vi "Set Channel PWM.vi"(8 "error in (no error)":errorcluster, 9 "PWM (0-255)":u8, 10 "LED Channel (0-18, 0=all)":u8=255, 11 "LINX-SN3218 in":refnum<class "LINX-SN3218.lvclass">) -> (0 "error out":errorcluster, 3 "LINX-SN3218 out":refnum<class "LINX-SN3218.lvclass">)   [LabVIEW 2020, in "LINX-SN3218.lvclass"]
doc: "Sets the individual PWM value (0-255 = 0-100% duty cycle) for the specified channel (0-18)."
uses:
  LINX-SN3218.lvclass
  LINX I2C/LINX I2C.lvclass
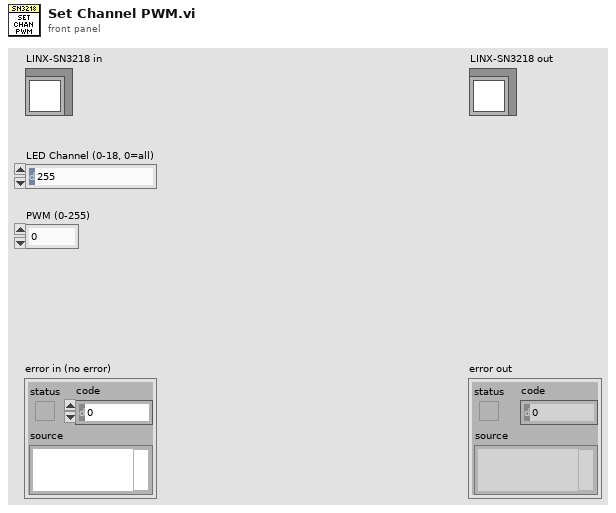
[diagram p1: front panel]
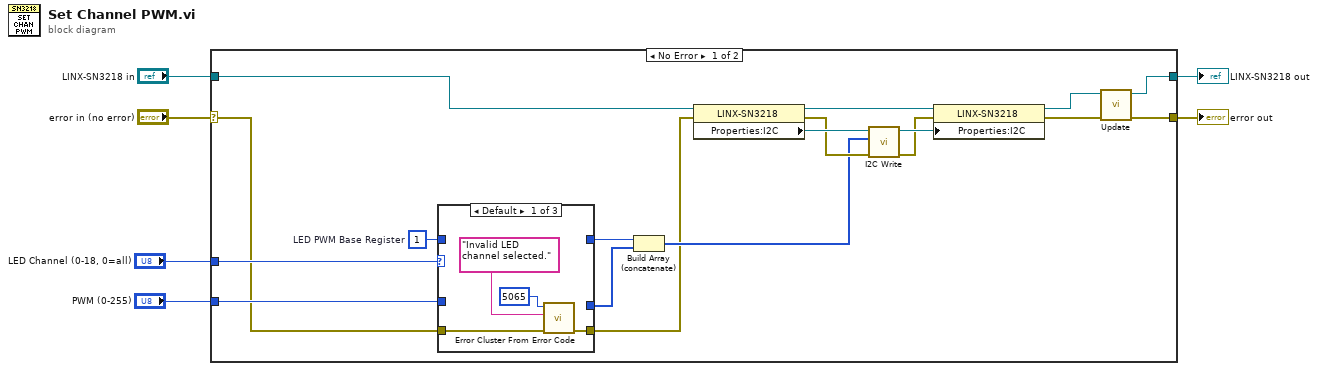
[diagram p0: block diagram]
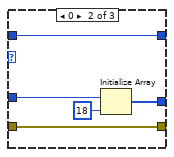
[diagram p2: hidden frame]
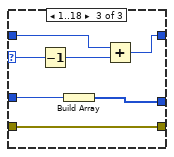
[diagram p3: hidden frame]
diagram:
  n1 = case shown="No Error" "error in (no error)" {
    selector: "error in (no error)" -> [w8 w42]
    tunnel: [w15 w42] -> w5
    tunnel: [w14 w41] -> w3
    tunnel: "LINX-SN3218 in" -> [w24 w41]
    tunnel: "LED Channel (0-18, 0=all)" -> [w12 _]
    tunnel: "PWM (0-255)" -> [w13 _]
    frame No Error {
      w10 = u8 1  # LED PWM Base Register
      n2 = case shown="Default" w12 {
        selector: w12 -> [_ _ w39]
        tunnel: w13 -> [_ w33 w36]
        tunnel: [_ w31 w35] -> w11
        tunnel: w10 -> [_ w30 w40]
        tunnel: [_ w30 w38] -> w9
        tunnel: w8 -> [w28 w29 w34]
        tunnel: [w27 w29 w34] -> w7
        frame Default {
          n3 = call <vilib>:"Error Cluster From Error Code.vi"("error in (no error)"=w28, "error message (\"\")"="Invalid LED channel selected.", "error code (0)"=5065) -> ("error out"=w27:errorcluster)  [unwired: 6 in]
        }
        frame 0 {
          n4 = Initialize Array(w33, 18 ("dimension size")) -> (w31:u8[])
        }
        frame 1..18 {
          n5 = Decrement(x=w39) -> (x-1=w37:u8)
          n6 = Build Array(w36) -> (w35:u8[])
          n7 = Add(x=w40, y=w37) -> (x+y=w38:u8)
        }
      }
      n8 = Build Array (concatenate)(w9, w11) -> (w18:u8[])
      n9 = property class="LINX-SN3218"(reference=w24, error in=w7) -> (reference out=w22:refnum<class "LINX-SN3218.lvclass">, error out=w20:errorcluster, "Properties:I2C"=w23:refnum<class "LINX I2C.lvclass">)
      n10 = call "I2C Write.vi"("error in (no error)"=w20, "Bytes to Write"=w18, "LINX I2C in"=w23) -> ("error out"=w19:errorcluster, "LINX I2C out"=w21:refnum<class "LINX I2C.lvclass">)  [unwired: 7 in]
      n11 = property class="LINX-SN3218"(reference=w22, error in=w19, "Properties:I2C"=w21) -> (reference out=w16:refnum<class "LINX-SN3218.lvclass">, error out=w17:errorcluster)
      n12 = call "Update.vi"("error in (no error)"=w17, "LINX-SN3218 in"=w16) -> ("error out"=w15:errorcluster, "LINX-SN3218 out"=w14:refnum<class "LINX-SN3218.lvclass">)  [unwired: 8 in]
    }
    frame Error {
    }
  }
  "error out" <- w5
  "LINX-SN3218 out" <- w3
